vi "ConcatArrayToCleanString.vi"(0 "stringArray":string[](array[string]), 1 "separator(;)":string=";") -> (2 "cleanDelimitedString":string)   [LabVIEW 2016]
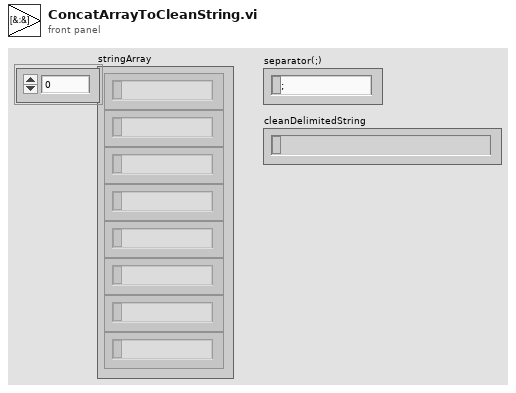
[diagram p1: front panel]
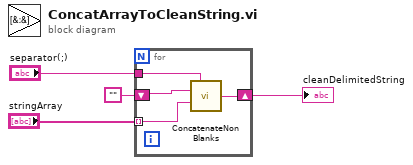
[diagram p0: block diagram]
diagram:
  n1 = for {
    tunnel: "stringArray" -> [w8] mode=indexing
    shift-right: [w7] -> w2
    shift-left: "" -> [w6]
    tunnel: "separator(;)" -> [w5]
    n2 = call "ConcatenateNonBlanks.vi"("separator"=w5, "prependString"=w6, "appendString"=w8) -> ("outputString"=w7:string)  [unwired: 12 in]
  }
  "cleanDelimitedString" <- w2
